vi "Actor Core.vi"(8 "error in":errorcluster, 11 "Nested in":refnum<class "Camera Prime95B Controller.lvclass">) -> (0 "error out":errorcluster, 3 "Actor out":refnum<class "Actor.lvclass">)   [LabVIEW 2020, in "Camera_Prime95B.lvlib" / "Camera Prime95B Controller.lvlib" / "Camera Prime95B Controller.lvclass"]
doc: "(<B>Filename</B>: Actor Framework.lvlib:Actor.lvclass:Actor Core.vi)\n\nReceives messages to the actor, reacts to them, and initiates any error handling that may shut the actor down.\n\nDescendant classes may override this VI to append parallel tasks for the actor to complete while it handles messages. Overrides use the Call Parent Method node."
uses:
  Camera Prime95B Controller.lvclass
  C:/Program Files/National Instruments/LabVIEW 2020/vi.lib/ActorFramework/Actor/Actor.lvclass
  <vilib>/ActorFramework/Actor/Actor.lvclass
  Camera Prime95B Controller.lvclass/Camera Prime95B Controller.ctl
  <vilib>/ActorFramework/Actor/Actor.lvclass/Actor.ctl
  <vilib>/ActorFramework/Message Enqueuer/Message Enqueuer.lvclass/Message Enqueuer.ctl
  Camera_Prime95B/Camera_Prime95B Messages/SetROI Msg/SetROI Msg.lvclass/SetROI Msg.ctl
  Camera_Prime95B/Camera_Prime95B Messages/StartSequenceAcqusition Msg/StartSequenceAcqusition Msg.lvclass/StartSequenceAcqusition Msg.ctl
  Camera_Prime95B/Camera_Prime95B/Acquisition Params.ctl
  Camera_Prime95B/Camera_Prime95B Messages/PreSequenceAcquisition Msg/PreSequenceAcquisition Msg.lvclass/PreSequenceAcquisition Msg.ctl
  Camera_Prime95B/Camera_Prime95B Messages/SetExposure Msg/SetExposure Msg.lvclass/SetExposure Msg.ctl
  Camera_Prime95B/Camera_Prime95B Messages/SetBinning Msg/SetBinning Msg.lvclass/SetBinning Msg.ctl
  <vilib>/ActorFramework/Message Enqueuer/Init from Existing Queue.vi
  <vilib>/ActorFramework/Message Enqueuer/Enqueue.vi
  Camera_Prime95B/Camera_Prime95B Messages/SetROI Msg/SetROI Msg.lvclass
  C:/Program Files/National Instruments/LabVIEW 2020/vi.lib/ActorFramework/Message/Message.lvclass
  Camera_Prime95B/Camera_Prime95B Messages/ClearROI Msg/ClearROI Msg.lvclass
  Camera_Prime95B/Camera_Prime95B Messages/StartSequenceAcqusition Msg/StartSequenceAcqusition Msg.lvclass
  Camera_Prime95B/Camera_Prime95B Messages/PreSequenceAcquisition Msg/PreSequenceAcquisition Msg.lvclass
  Camera_Prime95B/Camera_Prime95B Messages/StopSequenceAcqusition Msg/StopSequenceAcqusition Msg.lvclass
  <vilib>/ActorFramework/Stop Msg/Stop Msg.lvclass
  Camera_Prime95B/Camera_Prime95B Messages/SetExposure Msg/SetExposure Msg.lvclass
  Camera_Prime95B/Camera_Prime95B Messages/SetBinning Msg/SetBinning Msg.lvclass
  <vilib>/ActorFramework/Message Priority Queue/Priority Enqueue.vi
  <vilib>/ActorFramework/Message Enqueuer/Message Enqueuer.lvclass
  D:/Daguan/Development/MMicroscopyAF/Model/Real Hardware/Camera Prime95B Controller/Camera Prime95B Controller.lvclass
  Camera_Prime95B/Camera_Prime95B/Camera_Prime95B.lvclass
panel:
  in  "Save Path":path
  in  "Alert when finish?":bool
  in  "SingleStack?":bool
  in  "StreamToDisk?":bool
  in  "Binning":enum32{"1x1", "2x2"}(radio)
  in  "File suffix":string
  in  "Full":bool
  in  "Crop":bool
  in  "Scale Bar":bool
  in  "ScaleBarSize":dbl caption="um" min=0.0 max=50.0
  in  "FrameIndexSroll":i32(c297)
  in  "Save Settings":bool
  in  "Snap":bool
  in  "Live":bool
  in  "Acquire":bool
  in  "Stop":bool
  in  "Album":bool
  in  "Exit":bool
  in  "Interval":dbl min=0.0 max=99999.0
  in  "Frames":dbl min=0.0 max=5000.0
  in  "ExposureMs":dbl min=0.0 max=99999.0
  out "DropFrames":dbl
  out "RealFPS":dbl
  out "ImgIndex":dbl
  out "RawImage":T1(plugin-control)
  # "ROI"
  # "Save Image Mode"
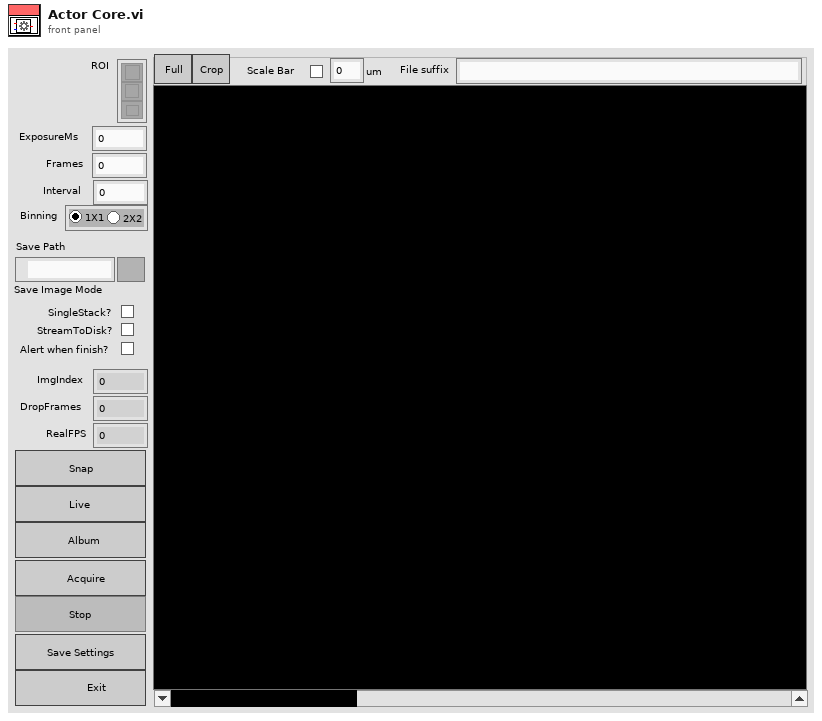
[diagram p1: front panel]
types:
  T1 = typedef "IMAQ Image.ctl" = refnum<image>
  T2 = cluster{"Stop":refnum<user-event>, "RawImage":refnum<user-event>}
  T3 = typedef "Camera_Prime95B.lvlib/Camera_Prime95B.lvclass/Acquisition Params.ctl" = cluster{"ExposureMs":dbl, "Frames":dbl, "Interval":dbl, "Save Path":path, "Stream Save Path":path, "SingleStack?":bool, "StreamToDisk?":bool, "Alert when finish?":bool, "File suffix":string}
  T4 = cluster{"Global Rectangle":i32[], "Contours":cluster{"Contour Type":u32, "ROI Type":u32, "Points":i32[]}[]}
  T5 = cluster{"Global Rectangle[0]":i32, "Global Rectangle[1]":i32, "Global Rectangle[2]":i32, "Global Rectangle[3]":i32}
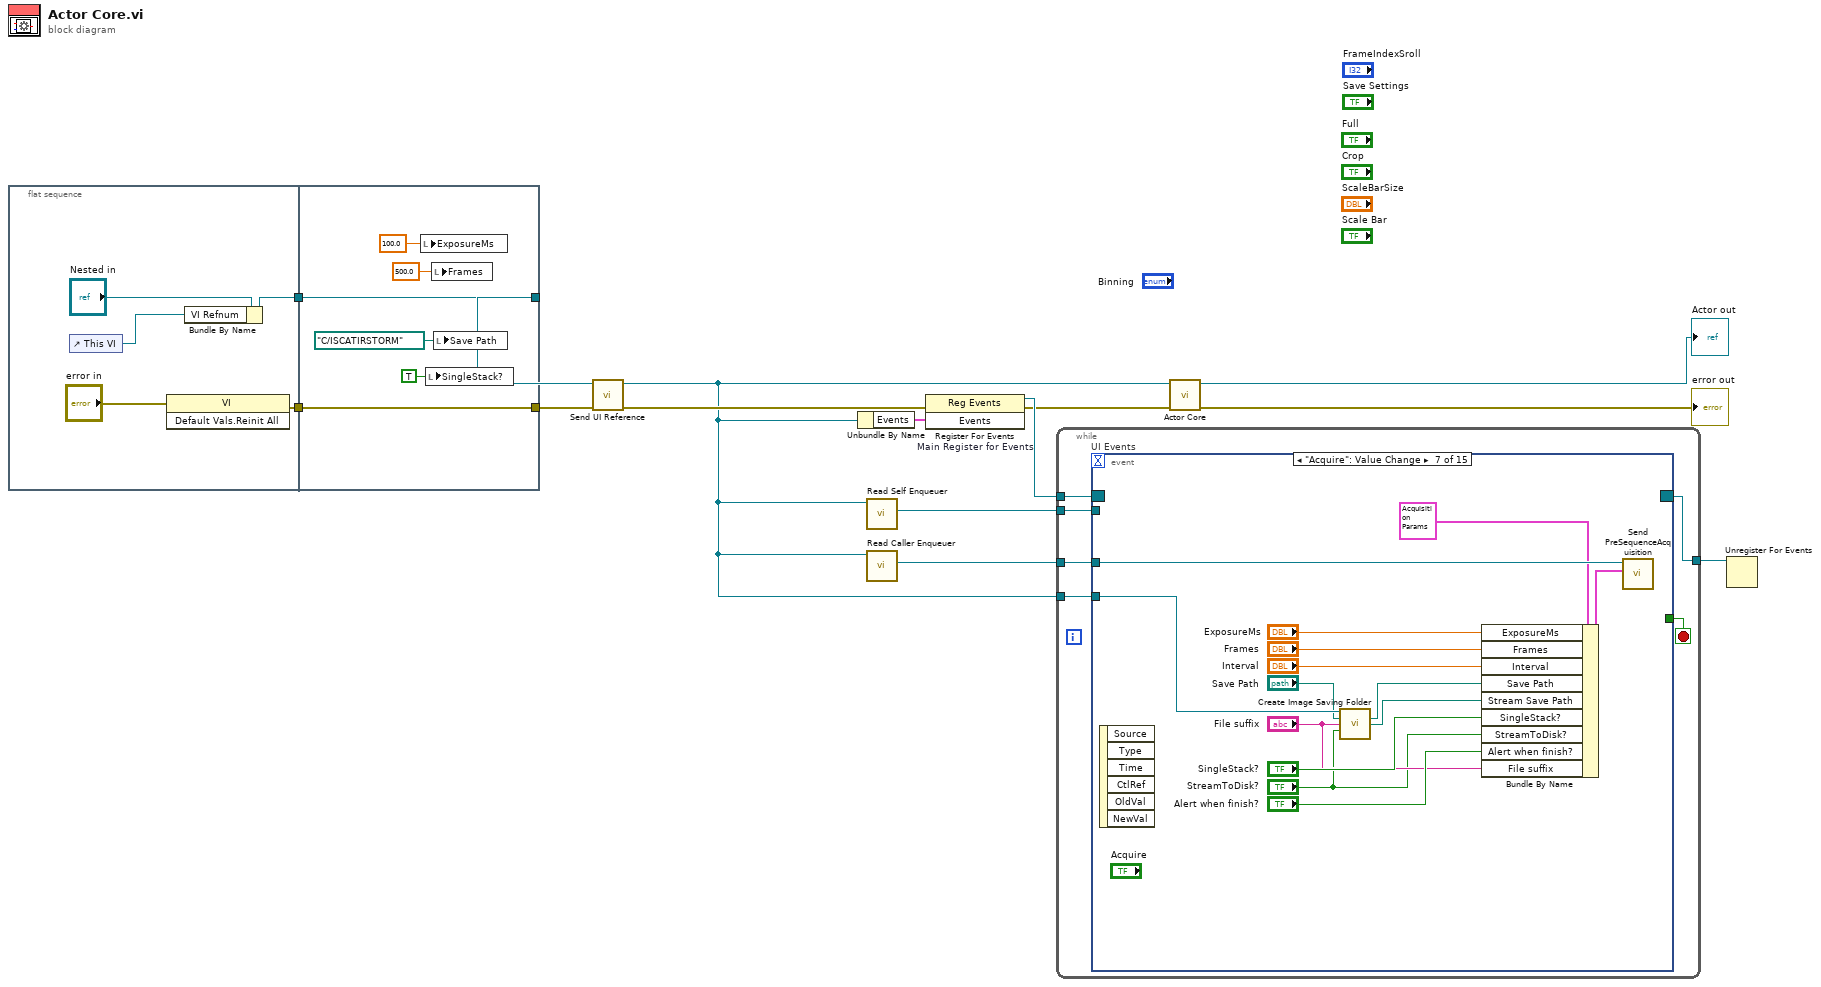
[diagram p0: block diagram]
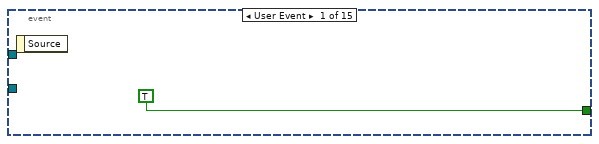
[diagram p2: hidden frame]
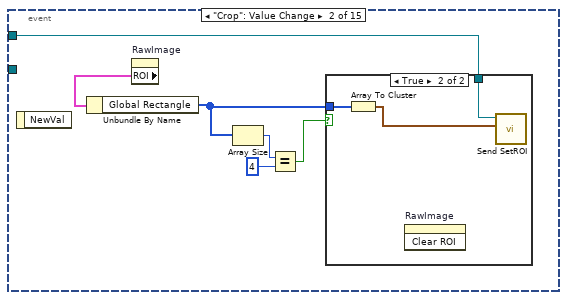
[diagram p3: hidden frame]
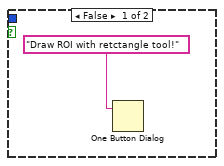
[diagram p4: hidden frame]
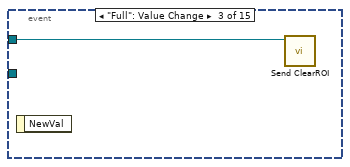
[diagram p5: hidden frame]
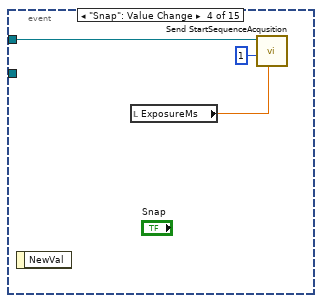
[diagram p6: hidden frame]
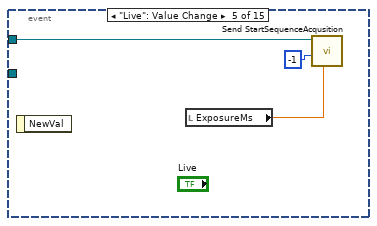
[diagram p7: hidden frame]
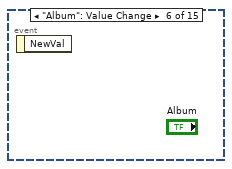
[diagram p8: hidden frame]
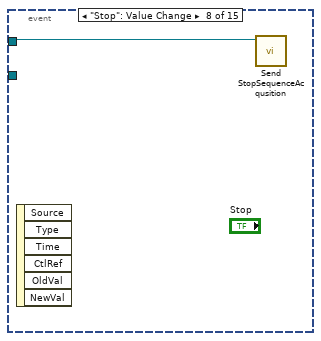
[diagram p9: hidden frame]
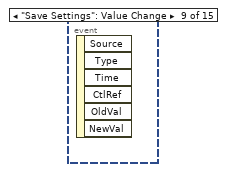
[diagram p10: hidden frame]
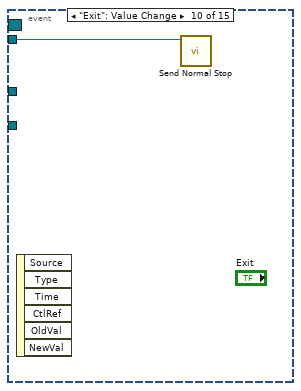
[diagram p11: hidden frame]
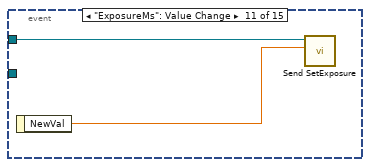
[diagram p12: hidden frame]
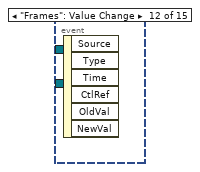
[diagram p13: hidden frame]
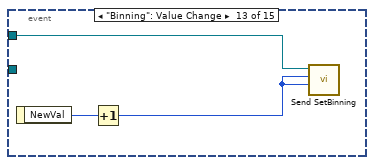
[diagram p14: hidden frame]
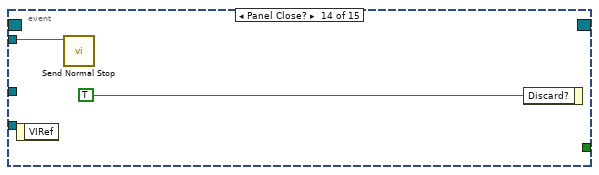
[diagram p15: hidden frame]
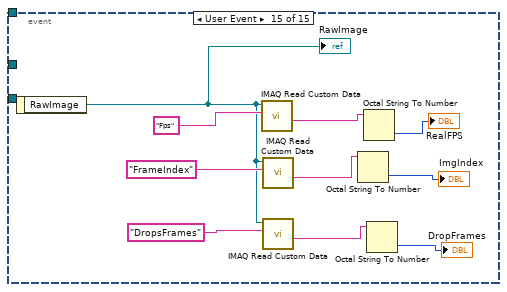
[diagram p16: hidden frame]
diagram:
  n1 = flat-sequence {
    tunnel: [w17] -> w6
    tunnel: [w16] -> w5
    tunnel: [w24] -> w2
    tunnel: [w25] -> w7
    tunnel: w6 -> [w25]
    tunnel: w5 -> [w24]
    frame #0 {
      n2 = control-ref of="This VI"() -> (w15:refnum<vi>)
      n3 = invoke class="VI" method="Default Vals.Reinit All"(error in="error in") -> (error out=w17:errorcluster)  [unwired: 2 in, 2 out]
      n4 = Bundle By Name(cluster="Nested in", "VI Refnum"=w15) -> (w16:refnum<class "Camera Prime95B Controller.lvclass">)
    }
    frame #1 {
      n5 = local write "ExposureMs"(100.0 ("ExposureMs")) -> ()
      n6 = local write "SingleStack?"(TRUE ("SingleStack?")) -> ()
      n7 = local write "Frames"(500.0 ("Frames")) -> ()
      n8 = local write "Save Path"(path "C:/ISCATIRSTORM" ("Save Path")) -> ()
    }
  }
  n9 = call-dynamic "Send UI Reference.vi"("error in (no error)"=w7, "Camera Prime95B Controller in"=w2) -> ("error out"=w3:errorcluster, "Camera Prime95B Controller out"=w1:refnum<class "Camera Prime95B Controller.lvclass">)  [unwired: 8 in]
  n10 = Unbundle By Name(w1) -> ("Events"=w11:T2)
  n11 = call <vilib>:"Read Self Enqueuer.vi"("Actor"=w1) -> ("Self Enqueuer"=w9:refnum<class "Message Enqueuer.lvclass">)  [unwired: 10 in]
  n12 = call <vilib>:"Read Caller Enqueuer.vi"("Actor"=w1) -> ("Caller Enqueuer"=w4:refnum<class "Message Enqueuer.lvclass">)  [unwired: 10 in]
  n13 = register-events "Main Register for Events"(error in=w3, w11) -> (reference out=w12:refnum<event-registration>, error out=w8:errorcluster)  [unwired: 1 in]
  n14 = while {
    tunnel: w12 -> [w31]
    tunnel: [w29] -> w10
    tunnel: w9 -> [w28]
    tunnel: w4 -> [w27]
    tunnel: w1 -> [w26]
    stop <- w30 stop-if-true
    n15 = event "UI Events" shown="[6] \"Acquire\": Value Change" {
      selector: w31 -> [_ _ _ _ _ _ _ _ _ _ _ _ _ _ _]
      dyn-events: [_ _ _ _ _ _ _ _ _ _ _ _ _ _ _] -> w29
      timeout: _ -> [_ _ _ _ _ _ _ _ _ _ _ _ _ _ _]
      tunnel: [TRUE _ _ _ _ _ _ _ _ _ _ _ _ _ _] -> w30
      tunnel: w28 -> [_ _ _ _ _ _ _ _ _ w65 _ _ _ w71 _]
      tunnel: w27 -> [_ w33 w43 w46 w47 _ w63 w64 _ _ w67 _ w70 _ _]
      tunnel: w26 -> [_ _ _ _ _ _ w55 _ _ _ _ _ _ _ _]
      event User Event {
        n16 = event-data() -> ()  [unwired: 1 in, 1 out]
      }
      event "Crop": Value Change {
        n17 = event-data() -> ()  [unwired: 1 in, 1 out]
        n18 = property on="RawImage" class="ImageControl"() -> ("ROI"=w38:T4)  [unwired: 2 in, 2 out]
        n19 = Unbundle By Name(w38) -> ("Global Rectangle"=w34:i32[])
        n20 = Array Size(array=w34) -> (size(s)=w37:i32)
        n21 = Equal?(x=w37, y=4) -> (x = y?=w35:bool)
        n22 = case shown="True" w35 {
          tunnel: w34 -> [_ w42]
          tunnel: w33 -> [_ w41]
          frame False {
            n23 = One Button Dialog(message="Draw ROI with retctangle tool!") -> ()  [unwired: 1 in, 1 out]
          }
          frame True {
            n24 = Array To Cluster(array=w42) -> (cluster=w40:T5)
            n25 = invoke on="RawImage" class="ImageControl" method="Clear ROI"() -> ()  [unwired: 3 in, 3 out]
            n26 = call "Send SetROI.vi"("Setting.ROI"=w40, "Message Enqueuer"=w41) -> ()  [unwired: 8 in, 2 out]
          }
        }
      }
      event "Full": Value Change {
        n27 = event-data() -> ()  [unwired: 1 in, 1 out]
        n28 = call "Send ClearROI.vi"("Message Enqueuer"=w43) -> ()  [unwired: 9 in, 2 out]
      }
      event "Snap": Value Change {
        n29 = event-data() -> ()  [unwired: 1 in, 1 out]
        n30 = local read "ExposureMs"() -> (w45:dbl)
        n31 = call "Send StartSequenceAcqusition.vi"("Exposure"=w45, "Frames"=1, "Message Enqueuer"=w46) -> ()  [unwired: 7 in, 2 out]
      }
      event "Live": Value Change {
        n32 = event-data() -> ()  [unwired: 1 in, 1 out]
        n33 = local read "ExposureMs"() -> (w49:dbl)
        n34 = call "Send StartSequenceAcqusition.vi"("Exposure"=w49, "Frames"=-1, "Message Enqueuer"=w47) -> ()  [unwired: 7 in, 2 out]
      }
      event "Album": Value Change {
        n35 = event-data() -> ()  [unwired: 1 in, 1 out]
      }
      event "Acquire": Value Change {
        n36 = event-data() -> ()  [unwired: 1 in, 6 out]
        n37 = call-dynamic "Create Image Saving Folder.vi"("Camera Prime95B Controller in"=w55, "Save Path"="Save Path", "File suffix"="File suffix", "StreamToDisk?"="StreamToDisk?") -> ("Saving Path"=w51:path, "Stream Saving Path"=w50:path)  [unwired: 8 in, 2 out]
        n38 = Bundle By Name(cluster=T3 {"ExposureMs"=0.0, "Frames"=0.0, "Interval"=0.0, "Save Path"=path "", "Stream Save Path"=path "", "SingleStack?"=FALSE, "StreamToDisk?"=FALSE, "Alert when finish?"=FALSE, "File suffix"=""} ("Acquisition Params"), "ExposureMs"="ExposureMs", "Frames"="Frames", "Interval"="Interval", "Save Path"=w51, "Stream Save Path"=w50, "SingleStack?"="SingleStack?", "StreamToDisk?"="StreamToDisk?", "Alert when finish?"="Alert when finish?", "File suffix"="File suffix") -> (w61:T3)
        n39 = call "Send PreSequenceAcquisition.vi"("Acquisition Params"=w61, "Message Enqueuer"=w63) -> ()  [unwired: 8 in, 2 out]
      }
      event "Stop": Value Change {
        n40 = event-data() -> ()  [unwired: 1 in, 6 out]
        n41 = call "Send StopSequenceAcqusition.vi"("Message Enqueuer"=w64) -> ()  [unwired: 9 in, 2 out]
      }
      event "Save Settings": Value Change {
        n42 = event-data() -> ()  [unwired: 1 in, 6 out]
      }
      event "Exit": Value Change {
        n43 = event-data() -> ()  [unwired: 1 in, 6 out]
        n44 = call <vilib>:"Send Normal Stop.vi"("Message Enqueuer"=w65) -> ()  [unwired: 10 in, 1 out]
      }
      event "ExposureMs": Value Change {
        n45 = event-data() -> ("NewVal"=w66:dbl)  [unwired: 1 in]
        n46 = call "Send SetExposure.vi"("Setting.Exposure"=w66, "Message Enqueuer"=w67) -> ()  [unwired: 8 in, 2 out]
      }
      event "Frames": Value Change {
        n47 = event-data() -> ()  [unwired: 1 in, 6 out]
      }
      event "Binning": Value Change {
        n48 = event-data() -> ("NewVal"=w69:enum32{"1x1", "2x2"})  [unwired: 1 in]
        n49 = Increment(x=w69) -> (x+1=w68:enum32{"1x1", "2x2"})
        n50 = call "Send SetBinning.vi"("Setting.Binning.BinY"=w68, "Setting.Binning.BinX"=w68, "Message Enqueuer"=w70) -> ()  [unwired: 7 in, 2 out]
      }
      event Panel Close? {
        n51 = event-data() -> ()  [unwired: 1 in, 1 out]
        n52 = call <vilib>:"Send Normal Stop.vi"("Message Enqueuer"=w71) -> ()  [unwired: 10 in, 1 out]
        n53 = event-data("Discard?"=TRUE) -> ()  [unwired: 1 in, 1 out]
      }
      event User Event {
        n54 = event-data() -> ("RawImage"=w80:T1)  [unwired: 1 in]
        "RawImage" <- w80
        n55 = call "IMAQ Read Custom Data"("Key"="Fps", "Image"=w80) -> ("Custom Data Out"=w78:string)  [unwired: 7 in, 2 out]
        n56 = call "IMAQ Read Custom Data"("Key"="FrameIndex", "Image"=w80) -> ("Custom Data Out"=w77:string)  [unwired: 7 in, 2 out]
        n57 = call "IMAQ Read Custom Data"("Key"="DropsFrames", "Image"=w80) -> ("Custom Data Out"=w76:string)  [unwired: 7 in, 2 out]
        n58 = Octal String To Number(4:w77) -> (0:→"ImgIndex":u32)  [unwired: 2 in, 1 out]
        n59 = Octal String To Number(4:w78) -> (0:→"RealFPS":u32)  [unwired: 2 in, 1 out]
        n60 = Octal String To Number(4:w76) -> (0:→"DropFrames":u32)  [unwired: 2 in, 1 out]
      }
    }
  }
  n61 = call-parent "Actor Core.vi"("error in"=w8, "Actor in"=w1) -> ("error out"=→"error out":errorcluster, "Actor out"=→"Actor out":refnum<class "Actor.lvclass">)  [unwired: 8 in]
  n62 = Unregister For Events(event registration refnum=w10) -> ()  [unwired: 1 in, 1 out]
